vi "Create Enum Metadata.vi"(8 "error in (no error)":errorcluster, 11 "ProtoFile Enums":u64[](array[numeric])) -> (0 "error out":errorcluster, 3 "Enum Parameters":T1[](array[typedef]))   [LabVIEW 2019, in "gRPC Template Creation Utility.lvlib"]
uses:
  gRPC Template Creation Utility.lvlib
  TypeDefs/Enum Metadata (Scripting).ctl
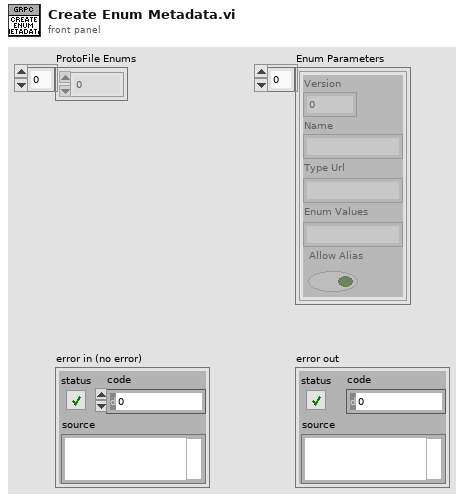
[diagram p1: front panel]
types:
  T1 = typedef "gRPC Template Creation Utility.lvlib/Enum Metadata (Scripting).ctl" = cluster{"Version":i32, "Name":string, "Type Url":string, "Enum Values":string, "Allow Alias":bool}
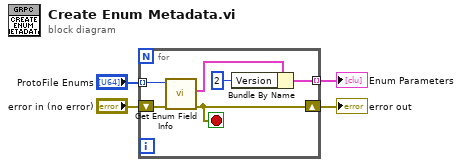
[diagram p0: block diagram]
diagram:
  n1 = for {
    tunnel: "ProtoFile Enums" -> [w7] mode=indexing
    shift-right: [w5] -> w4
    shift-left: "error in (no error)" -> [w8]
    tunnel: [w10] -> w1 mode=indexing
    stop <- w5 stop-if-true
    n2 = call "Get Enum Field Info.vi"("error in (no error)"=w8, "Enum Field ref in"=w7) -> ("error out"=w5:errorcluster, "Field Info"=w6:T1)  [unwired: 7 in, 1 out]
    n3 = Bundle By Name(cluster=w6, "Version"=2) -> (w10:T1)
  }
  "error out" <- w4
  "Enum Parameters" <- w1
